vi "writeFileHeaders.vi"(8 "error in (no error)":errorcluster, 11 "Logger in":refnum<class "Logger.lvclass">) -> (0 "error out":errorcluster, 3 "Logger out":refnum<class "Logger.lvclass">)   [LabVIEW 2013, in "Logger.lvclass"]
uses:
  Logger.lvclass
  Logger.lvclass/Logger.ctl
  <vilib>/Utility/file.llb/Write To Spreadsheet File (string).vi
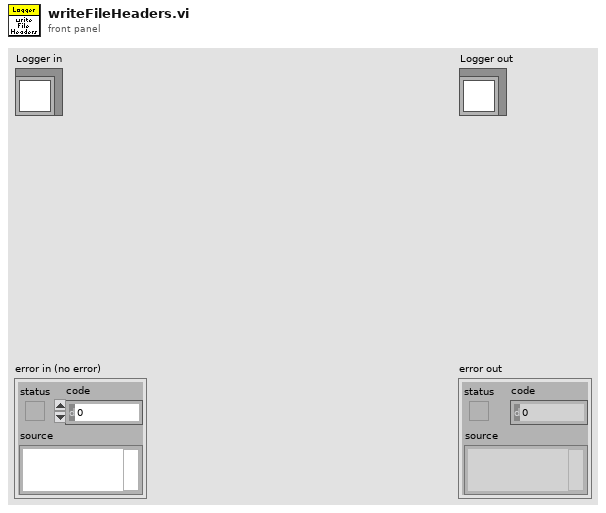
[diagram p1: front panel]
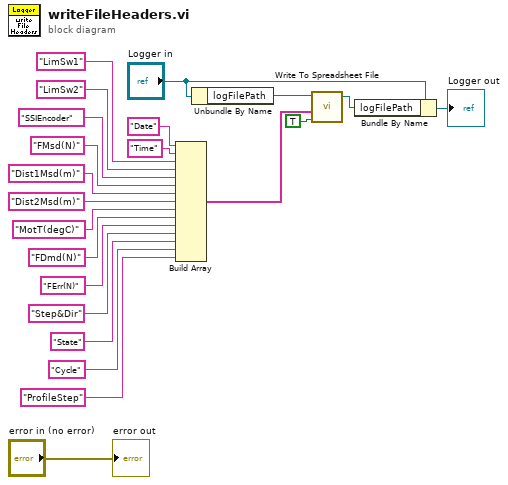
[diagram p0: block diagram]
diagram:
  n1 = Build Array("Date" ("element"), "Time", "LimSw1", "LimSw2", "SSIEncoder", "FMsd(N)", "Dist1Msd(m)", "Dist2Msd(m)", "MotT(degC)", "FDmd(N)", "FErr(N)", "Step&Dir", "State", "Cycle", "ProfileStep") -> (w4:string[])
  n2 = Unbundle By Name("Logger in") -> ("logFilePath"=w2:path)
  n3 = call-poly <vilib>:"Write To Spreadsheet File.vi"("append to file? (new file:F)"=TRUE, "1D data"=w4, "file path (dialog if empty)"=w2) -> ("new file path (Not A Path if cancelled)"=w5:path)  [unwired: 5 in]
  n4 = Bundle By Name(cluster="Logger in", "logFilePath"=w5) -> (→"Logger out":refnum<class "Logger.lvclass">)
  "error out" <- "error in (no error)"
